vi "Example Callback.vi"() -> ()   [LabVIEW 2010]
uses:
  C:/tf/play/labview/Tinkerforge.dll
  Tinkerforge.dll
panel:
  in  "stop":bool
  out "distance (cm)":i32
  in  "uid":string="amb"
  in  "port":i32=4223
  in  "host":string="localhost"
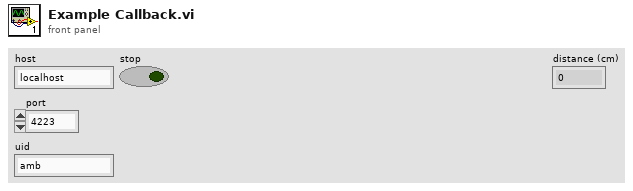
[diagram p1: front panel]
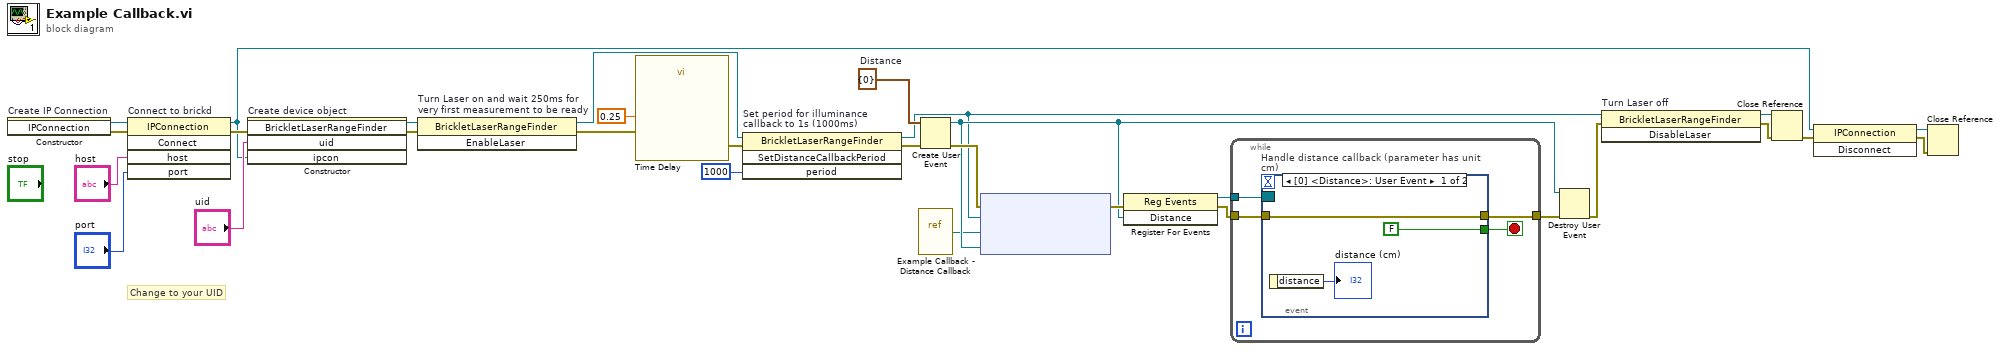
[diagram p0: block diagram]
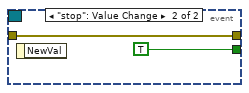
[diagram p2: hidden frame]
diagram:
  w15 = cluster{"distance":i32} {"distance"=0}  # Distance
  # "Change to your UID"
  n1 = constructor on="Create IP Connection" class="IPConnection"() -> (reference out=w30:refnum<k24>, error out=w12:errorcluster)  [unwired: 3 in, 1 out]
  n2 = invoke on="Connect to brickd" class="IPConnection" method="Connect"(reference=w30, error in=w12, "host"="host", "port"="port") -> (reference out=w23:refnum<k24>, error out=w26:errorcluster)  [unwired: 1 in, 3 out]
  n3 = constructor on="Create device object" class="BrickletLaserRangeFinder"(error in=w26, "uid"="uid", "ipcon"=w23) -> (reference out=w6:refnum<k24>, error out=w7:errorcluster)  [unwired: 2 in, 3 out]
  n4 = invoke on="Turn Laser on and wait 250ms for\nvery first measurement to be ready" class="BrickletLaserRangeFinder" method="EnableLaser"(reference=w6, error in=w7) -> (reference out=w8:refnum<k24>, error out=w9:errorcluster)  [unwired: 1 in, 1 out]
  n5 = call "Time Delay"("error in (no error)"=w9, "Delay Time (s)"=0.25) -> ("error out"=w10:errorcluster)  [unwired: 9 in]
  n6 = invoke on="Set period for illuminance\ncallback to 1s (1000ms)" class="BrickletLaserRangeFinder" method="SetDistanceCallbackPeriod"(reference=w8, error in=w10, "period"=i64 1000) -> (reference out=w3:refnum<k24>, error out=w14:errorcluster)  [unwired: 1 in, 2 out]
  n7 = vi-ref "Example Callback - Distance Callback.vi"() -> ("vi reference"=w1:refnum<vi>)
  n8 = Create User Event(user event datatype=w15, error in=w14) -> (user event=w16:refnum<user-event>, error out=w21:errorcluster)
  n9 = node ("Register Event Callback")(w21, w3, w1, w16) -> (w20:errorcluster)  [unwired: 1 in, 1 out]
  n10 = register-events(error in=w20, w16) -> (reference out=w19:refnum<event-registration>, error out=w17:errorcluster)  [unwired: 1 in]
  n11 = while {
    tunnel: w19 -> [w34]
    tunnel: [w33] -> w18
    tunnel: w17 -> [w32]
    stop <- w31 stop-if-true
    n12 = event "Handle distance callback (parameter has unit cm)" shown="[0] <Distance>: User Event" {
      selector: w34 -> [_ _]
      dyn-events: _ -> [_ _]
      timeout: _ -> [_ _]
      tunnel: [w37 w38] -> w33
      tunnel: w32 -> [w37 w38]
      tunnel: [FALSE TRUE] -> w31
      event User Event {
        n13 = event-data() -> ("distance"=→"distance (cm)":i32)  [unwired: 1 in]
      }
      event "stop": Value Change {
        n14 = event-data() -> ()  [unwired: 1 in, 1 out]
      }
    }
  }
  n15 = Destroy User Event(user event=w16, error in=w18) -> (error out=w5:errorcluster)
  n16 = invoke on="Turn Laser off" class="BrickletLaserRangeFinder" method="DisableLaser"(reference=w3, error in=w5) -> (reference out=w2:refnum<k24>, error out=w4:errorcluster)  [unwired: 1 in, 1 out]
  n17 = Close Reference(reference=w2, error in (no error)=w4) -> (error out=w25:errorcluster)
  n18 = invoke class="IPConnection" method="Disconnect"(reference=w23, error in=w25) -> (reference out=w22:refnum<k24>, error out=w24:errorcluster)  [unwired: 1 in, 1 out]
  n19 = Close Reference(reference=w22, error in (no error)=w24) -> ()  [unwired: 1 out]
